vi "Structures General.vi"() -> ()   [LabVIEW 2022 SP3]
panel:
  out "number (0 to 1)":dbl
  out "x*y":dbl
  in  "stop":bool
  in  "Enum":enum16{"C", "B", "A"}(ring)
  in  "Boolean":bool
  out "Numeric 7":dbl
  in  "Numeric 6":dbl
  in  "Numeric 5":dbl
  out "Numeric 4":dbl
  in  "Numeric 3":dbl
  in  "Numeric 2":dbl
  out "Numeric":i32
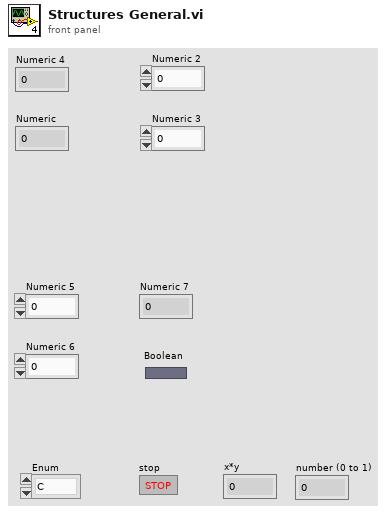
[diagram p1: front panel]
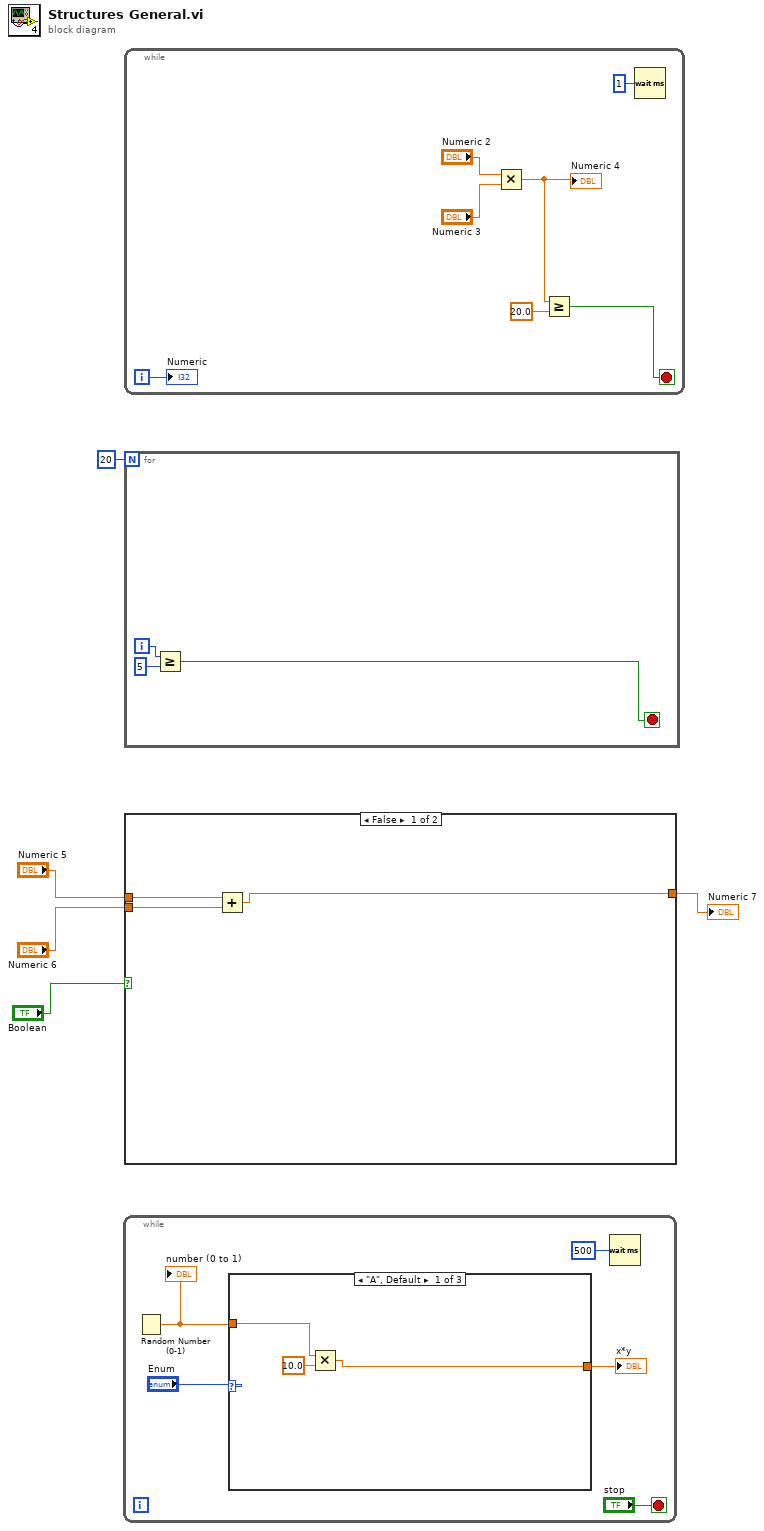
[diagram p0: block diagram]
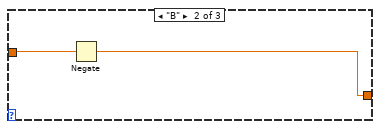
[diagram p2: hidden frame]
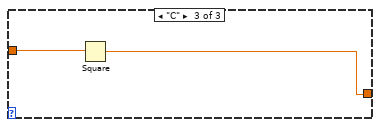
[diagram p3: hidden frame]
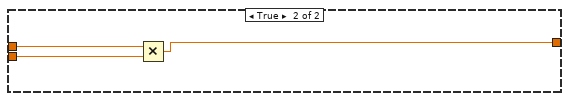
[diagram p4: hidden frame]
diagram:
  n1 = while {
    stop <- "stop" stop-if-true
    n2 = Random Number (0-1)() -> (number: 0 to 1=w8:dbl)
    "number (0 to 1)" <- w8
    n3 = case shown="\"A\", Default" "Enum" {
      tunnel: w8 -> [w13 w15 w17]
      tunnel: [w11 w14 w16] -> w7
      frame "A", Default {
        n4 = Multiply(x=w13, y=10.0) -> (x*y=w11:dbl)
      }
      frame "B" {
        n5 = Negate(x=w15) -> (-x=w14:dbl)
      }
      frame "C" {
        n6 = Square(x=w17) -> (x^2=w16:dbl)
      }
    }
    "x*y" <- w7
    n7 = Wait (ms)(milliseconds to wait=u32 500 ("millisecond timer value")) -> ()  [unwired: 1 out]
  }
  n8 = while {
    i -> [w23]
    stop <- w18 stop-if-true
    n9 = Multiply(x="Numeric 2", y="Numeric 3") -> (x*y=w19:dbl)
    "Numeric 4" <- w19
    n10 = Greater Or Equal?(x=w19, y=20.0) -> (x >= y?=w18:bool)
    n11 = Wait (ms)(milliseconds to wait=u32 1) -> ()  [unwired: 1 out]
    "Numeric" <- w23
  }
  n12 = for {
    N: 20 -> [_]
    i -> [w27]
    stop <- w25 stop-if-true
    n13 = Greater Or Equal?(x=w27, y=5) -> (x >= y?=w25:bool)
  }
  n14 = case shown="False" "Boolean" {
    tunnel: "Numeric 5" -> [w30 w33]
    tunnel: "Numeric 6" -> [w29 w32]
    tunnel: [w28 w31] -> w2
    frame False {
      n15 = Add(x=w30, y=w29) -> (x+y=w28:dbl)
    }
    frame True {
      n16 = Multiply(x=w33, y=w32) -> (x*y=w31:dbl)
    }
  }
  "Numeric 7" <- w2
